vi "TreeCtrl.vi"(8 "错误输入（无错误）":errorcluster, 10 "Vibration Channel Name":string[](array[string]), 11 "Tree in":refnum<vi>) -> (0 "错误输出":errorcluster)   [LabVIEW 2011]
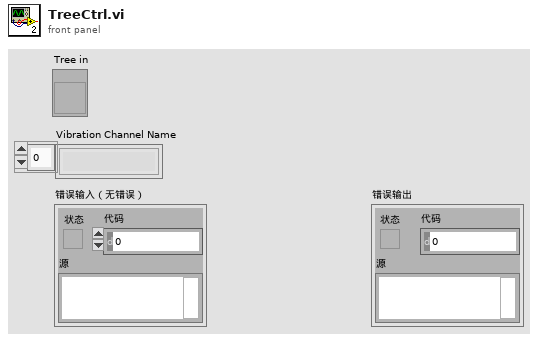
[diagram p1: front panel]
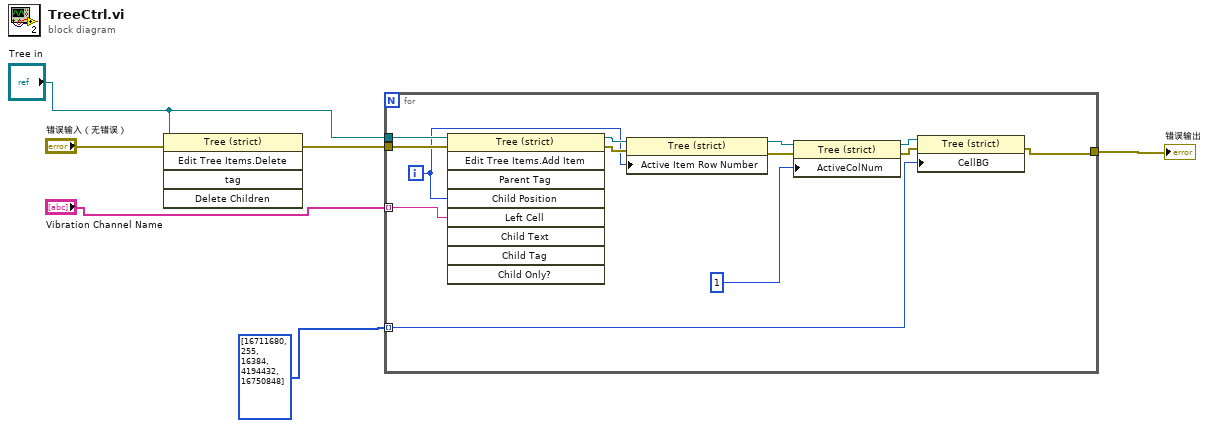
[diagram p0: block diagram]
diagram:
  n1 = invoke on="调用节点" class="Tree (strict)" method="Edit Tree Items.Delete"(reference="Tree in", error in="错误输入（无错误）") -> (error out=w6:errorcluster)  [unwired: 3 in, 4 out]
  n2 = for {
    tunnel: w6 -> [w19]
    tunnel: "Tree in" -> [w18]
    tunnel: "Vibration Channel Name" -> [w17] mode=indexing
    tunnel: u32[] [16711680, 255, 16384, 4194432, 16750848] -> [w13] mode=indexing
    tunnel: [w7] -> w2
    i -> [w8]
    n3 = invoke on="调用节点" class="Tree (strict)" method="Edit Tree Items.Add Item"(reference=w18, error in=w19, "Child Position"=w8, "Left Cell"=w17) -> (reference out=w12:refnum<vi>, error out=w10:errorcluster)  [unwired: 5 in, 7 out]
    n4 = property class="Tree (strict)"(reference=w12, error in=w10, "Active Item Row Number"=w8) -> (reference out=w11:refnum<vi>, error out=w9:errorcluster)
    n5 = property class="Tree (strict)"(reference=w11, error in=w9, "ActiveColNum"=1 ("活动单元格:活动列数")) -> (reference out=w15:refnum<vi>, error out=w14:errorcluster)
    n6 = property class="Tree (strict)"(reference=w15, error in=w14, "CellBG"=w13) -> (error out=w7:errorcluster)  [unwired: 1 out]
  }
  "错误输出" <- w2
